vi "write hist cluster element.vi"(5 "Secondary":i32=-1, 7 "Primary":i32=-1, 8 "error in (no error)":errorcluster, 10 "histogram":T2 {"S:" format="%_3f"}, 11 "Hist cluster":T1) -> (0 "error out":errorcluster, 3 "Hist cluster":T1)   [LabVIEW 2016]
uses:
  Typedefs/Coincidence histogram cluster refnum.ctl
  Typedefs/Coincidence single histogram.ctl
panel:
  # "Leave Primary and Secondary unwired to use the channel indexes\nin the supplied histogram."
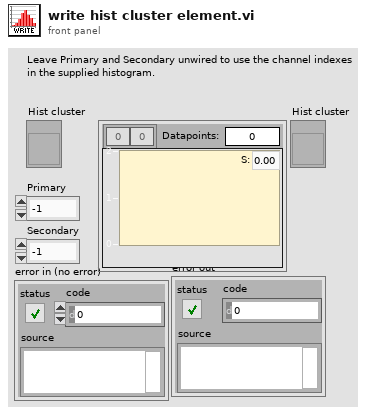
[diagram p1: front panel]
types:
  T1 = typedef "Coincidence histogram cluster refnum.ctl" = refnum<vi>
  T2 = typedef "Coincidence single histogram.ctl" = cluster{"Histogram Graph":cluster{"X Values":dbl[], "Histogram: h(x)":i32[]}[], "IDs":i8[], "Datapoints:":i32, "S:":dbl, "Data array":cluster{"Data":i32[], "Max index":i32, "Current index":i32, "Numofpoints":i32}}
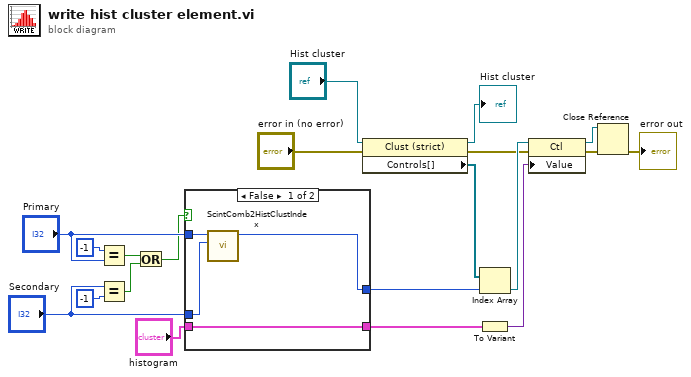
[diagram p0: block diagram]
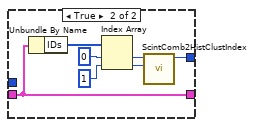
[diagram p2: hidden frame]
diagram:
  n1 = Equal?(x=-1, y="Primary") -> (x = y?=w3:bool)
  n2 = Equal?(x="Secondary", y=-1 ("x")) -> (x = y?=w4:bool)
  n3 = Or(x=w3, y=w4) -> (x .or. y?=w5:bool)
  n4 = case shown="False" w5 {
    tunnel: "Primary" -> [w24 _]
    tunnel: "Secondary" -> [w23 _]
    tunnel: [w22 w25] -> w10
    tunnel: [w21 w31] -> w1
    tunnel: "histogram" -> [w21 w31]
    frame False {
      n5 = call "ScintComb2HistClustIndex.vi"("Secondary"=w23, "Primary"=w24) -> ("Numeric"=w22:i32)  [unwired: 9 in]
    }
    frame True {
      n6 = Unbundle By Name(w31) -> ("IDs"=w30:i8[])
      n7 = Index Array(array=w30, index #1=0 ("index"), index #2=1 ("index")) -> (element #1=w27:i8, element #2=w26:i8)
      n8 = call "ScintComb2HistClustIndex.vi"("Secondary"=w26, "Primary"=w27) -> ("Numeric"=w25:i32)  [unwired: 9 in]
    }
  }
  n9 = property class="Clust (strict)"(reference="Hist cluster", error in="error in (no error)") -> (reference out=→"Hist cluster":T1, error out=w11:errorcluster, "Controls[]"=w19:refnum<vi>[])
  n10 = Index Array(array=w19, index=w10) -> (element=w12:refnum<vi>)
  n11 = To Variant(anything=w1) -> (Variant=w15:variant)
  n12 = property class="Ctl"(reference=w12, error in=w11, "Value"=w15) -> (reference out=w16:refnum<vi>, error out=w17:errorcluster)
  n13 = Close Reference(reference=w16, error in (no error)=w17) -> (error out=→"error out":errorcluster)
